vi "NET_PCM_Status.vi"(8 "Read(F) Write(T)":bool, 11 "PCM_Status_In":T1) -> (3 "PCM_Status_Out":T1)   [LabVIEW 2016]
uses:
  RoboRio code/TypeDef/CLUSTER_PCM_Status.ctl
  <vilib>/Rock Robotics/Network Tables/NT Write Boolean Array.vi
  <vilib>/Rock Robotics/Network Tables/NT Write Boolean.vi
  <vilib>/Rock Robotics/Network Tables/NT Write Numeric Array.vi
  <vilib>/Rock Robotics/Network Tables/NT Read Boolean Array.vi
  <vilib>/Rock Robotics/Network Tables/NT Read Boolean.vi
  <vilib>/Rock Robotics/Network Tables/NT Read Numeric Array.vi
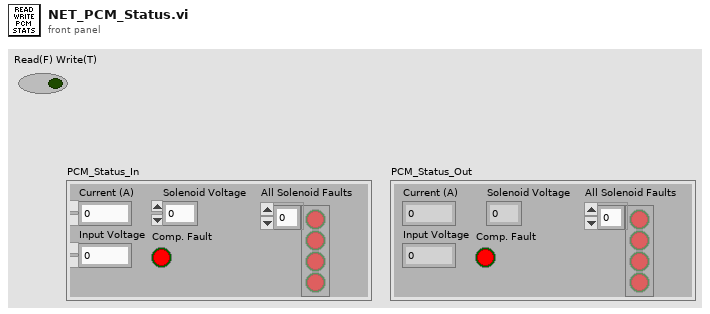
[diagram p1: front panel]
types:
  T1 = typedef "CLUSTER_PCM_Status.ctl" = cluster{"Current (A)":dbl, "All Solenoid Faults":bool[], "Input Voltage":dbl, "Solenoid Voltage":dbl, "Comp. Fault":bool}
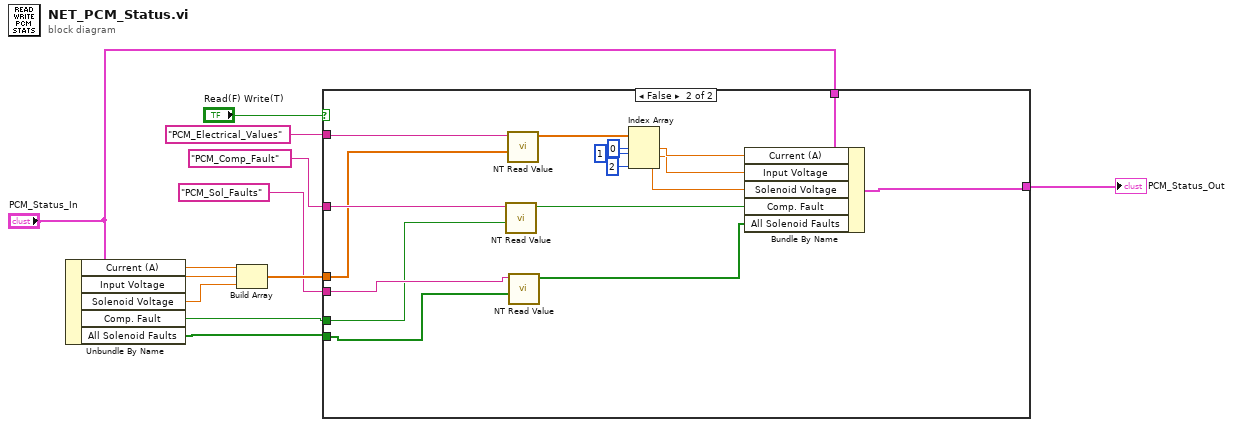
[diagram p0: block diagram]
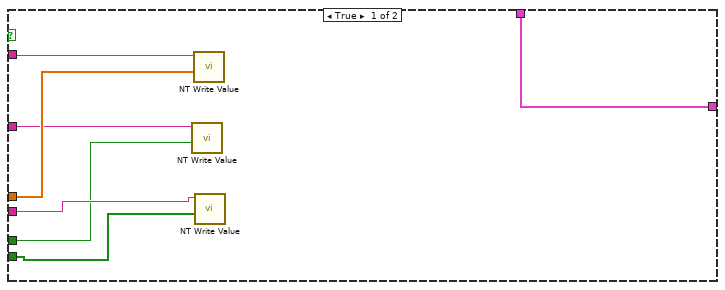
[diagram p2: hidden frame]
diagram:
  n1 = Unbundle By Name("PCM_Status_In") -> ("Current (A)"=w10:dbl, "Input Voltage"=w9:dbl, "Solenoid Voltage"=w8:dbl, "Comp. Fault"=w4:bool, "All Solenoid Faults"=w1:bool[])
  n2 = Build Array(w10, w9, w8) -> (w6:dbl[])
  n3 = case shown="False" "Read(F) Write(T)" {
    tunnel: "PCM_Electrical_Values" ("Name") -> [w17 w35]
    tunnel: [w14 w20] -> w2
    tunnel: "PCM_Comp_Fault" ("Name") -> [w16 w34]
    tunnel: w6 -> [w19 w31]
    tunnel: "PCM_Sol_Faults" ("Name") -> [w15 w33]
    tunnel: w1 -> [w18 w36]
    tunnel: "PCM_Status_In" -> [w14 w30]
    tunnel: w4 -> [w13 w32]
    frame True {
      n4 = call-poly <vilib>:"NT Write Value.vi"("Boolean"=w13, "Name"=w16) -> ()  [unwired: 9 in, 1 out]
      n5 = call-poly <vilib>:"NT Write Value.vi"("Numeric Array"=w19, "Name"=w17) -> ()  [unwired: 9 in, 1 out]
      n6 = call-poly <vilib>:"NT Write Value.vi"("Boolean Array"=w18, "Name"=w15) -> ()  [unwired: 9 in, 1 out]
    }
    frame False {
      n7 = call-poly <vilib>:"NT Read Value.vi"("Default Value"=w32, "Name"=w34) -> ("Boolean"=w22:bool)  [unwired: 8 in, 1 out]
      n8 = call-poly <vilib>:"NT Read Value.vi"("Default Value"=w31, "Name"=w35) -> ("Numeric Array"=w29:dbl[])  [unwired: 8 in, 1 out]
      n9 = call-poly <vilib>:"NT Read Value.vi"("Default Value"=w36, "Name"=w33) -> ("Boolean Array"=w21:bool[])  [unwired: 8 in, 1 out]
      n10 = Index Array(array=w29, index #1=0 ("index"), index #2=1 ("index"), index #3=2 ("index")) -> (element #1=w25:dbl, element #2=w24:dbl, element #3=w23:dbl)
      n11 = Bundle By Name(cluster=w30, "Current (A)"=w25, "Input Voltage"=w24, "Solenoid Voltage"=w23, "Comp. Fault"=w22, "All Solenoid Faults"=w21) -> (w20:T1)
    }
  }
  "PCM_Status_Out" <- w2
